vi "Status Status Info.vi"(8 "error in (no error)":errorcluster, 11 "VISA Resource in":refnum<visa-resource-name>) -> (0 "error out":errorcluster, 1 "Voltage (mV)":dbl, 2 "Restart Reason":string, 3 "VISA Resource out":refnum<visa-resource-name>)   [LabVIEW 2020, in "plugin_flodx_ph_probe.lvlib" / "mock_driver.lvlib"]
doc: "Emulates querying the status of the pH probe, but always returns the restart code \"P\" and a voltage of 5.038 mV."
uses:
  mock_driver.lvlib
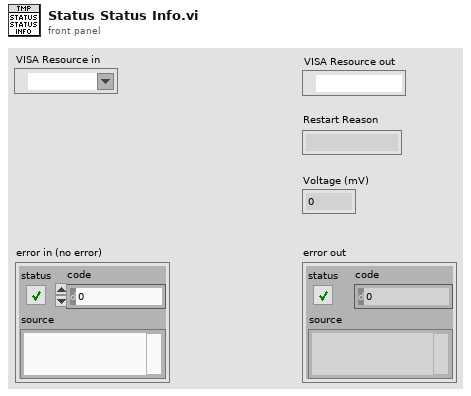
[diagram p1: front panel]
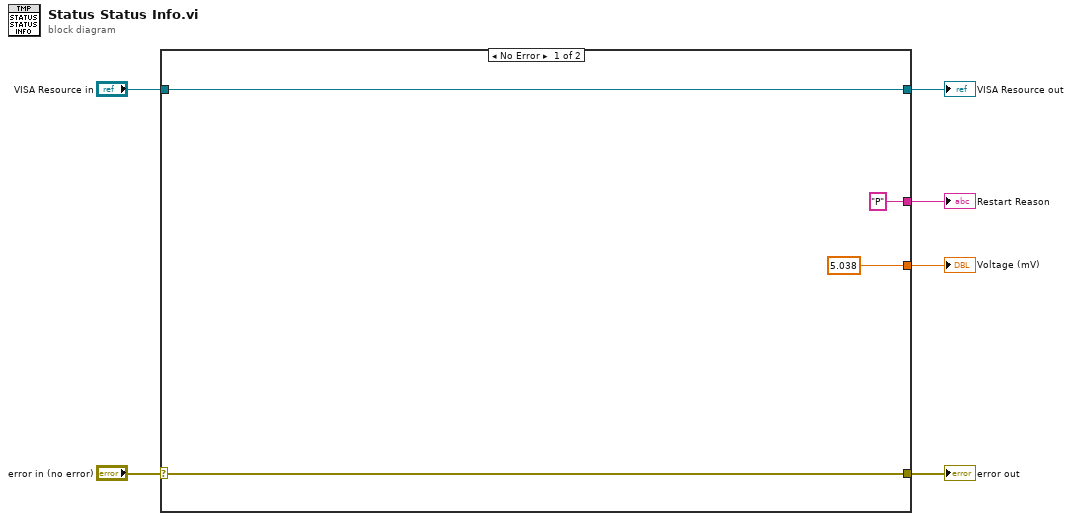
[diagram p0: block diagram]
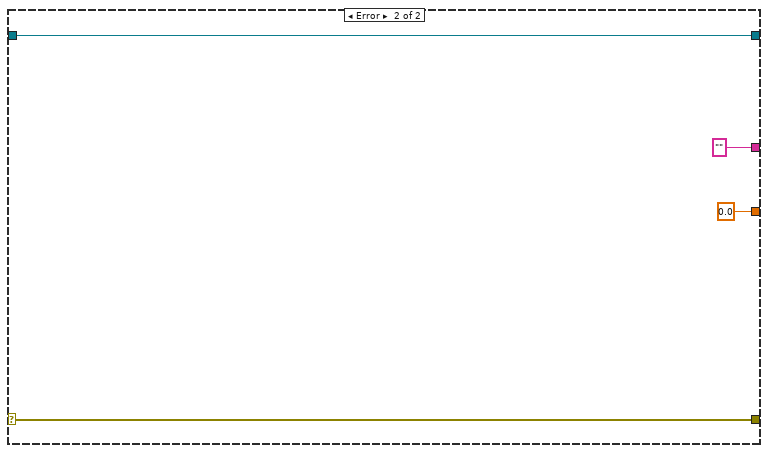
[diagram p2: hidden frame]
diagram:
  n1 = case shown="No Error" "error in (no error)" {
    selector: "error in (no error)" -> [w9 w13]
    tunnel: "VISA Resource in" -> [w10 w14]
    tunnel: [w10 w14] -> w5
    tunnel: [w9 w13] -> w3
    tunnel: [5.038 ("pH") 0.0 ("pH")] -> w2
    tunnel: ["P" ("Restart Reason") "" ("Restart Reason")] -> w1
    frame No Error {
    }
    frame Error {
    }
  }
  "VISA Resource out" <- w5
  "error out" <- w3
  "Voltage (mV)" <- w2
  "Restart Reason" <- w1
